vi "MCL Strings.vi"(8 "error in (no error)":errorcluster, 11 "Valve Item in":refnum<class "Valve Item.lvclass">) -> (0 "error out":errorcluster, 2 "Multicolumn Listxox row strings":string[](array[string]), 3 "Valve Item out":refnum<class "Valve Item.lvclass">)   [LabVIEW 2020, in "BetterDragAndDropDemo.lvlib" / "Valve Item.lvclass"]
uses:
  Valve Item.lvclass
  Valve Item.lvclass/Valve Item.ctl
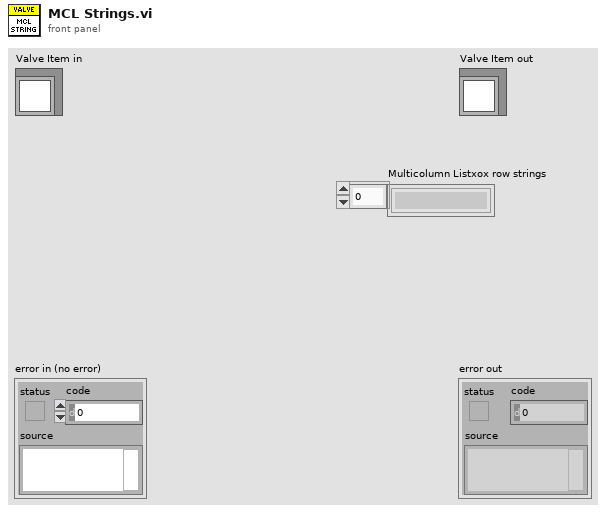
[diagram p1: front panel]
types:
  T1 = typedef "BetterDragAndDropDemo.lvlib/Valve Item.lvclass/valve color.ctl" = enum16{"black", "red"}
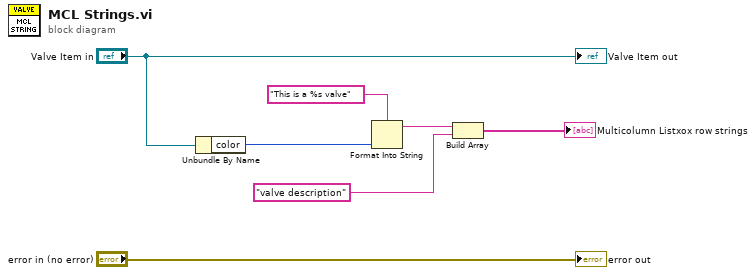
[diagram p0: block diagram]
diagram:
  n1 = Unbundle By Name("Valve Item in") -> ("color"=w5:T1)
  n2 = Format Into String(format string="This is a %s valve", w5) -> (resulting string=w3:string)  [unwired: 2 in, 1 out]
  n3 = Build Array(w3, "valve description" ("String")) -> (→"Multicolumn Listxox row strings":string[])
  "error out" <- "error in (no error)"
  "Valve Item out" <- "Valve Item in"
